vi "GUI_laptop v12.vi"() -> ()   [LabVIEW 2019]
uses:
  <vilib>/Math Plots/3D Math Plots/3D Scatter/3D Scatter XCtrl/3D Scatter.xctl
  <vilib>/Platform/TimedLoop/XDataNode/timing_clust.ctl
  <vilib>/Platform/TimedLoop/XDataNode/nitl_modes.ctl
  <vilib>/Platform/TimedLoop/XDataNode/wakeup.ctl
  <vilib>/Analysis/_algsub.llb/Real Vector Norm.vi
  <vilib>/Instr/_visa.llb/VISA Configure Serial Port (Instr).vi
  <vilib>/Utility/file.llb/Write Delimited Spreadsheet (DBL).vi
  <vilib>/Math Plots/3D Math Plots/3D Scatter/3D Scatter Datatype/Public/Plot Helper (Vector).vi
  <vilib>/platform/TimedLoop/XDataNode/XDataNode.xnode
  <vilib>/Platform/TimedLoop/XDataNode/XDNodeRunTimeDep.lvlib
  <vilib>/Analysis/NI_AALPro.lvlib
  <vilib>/Math Plots/3D Math Plots/3D Scatter/3D Scatter Datatype/3D Scatter Datatype.lvclass
panel:
  out "Numeric":i32
  out "send values":dbl[](array[numeric])
  out "Robot Feedback (xyz)":dbl[](array[numeric])
  in  "UDP Send":bool
  in  "UDP Recv":bool
  in  "L5 bound":dbl=1000.0
  in  "L4 bound (deg)":dbl=1000.0
  in  "L3 bound (mm)":dbl=1000.0
  in  "L2 bound (deg)":dbl=1000.0
  in  "L1 bound (deg)":dbl=1000.0
  in  "Joystick Type":dbl(ring) items=["Rigid Joystick", "Free Joystick"]
  out "Finished Late? [i-1]":bool
  in  "Epsilon":dbl=0.2
  out "3D Scatter":refnum<class "3D Plot Datatype.lvclass">[](xcontrol)
  out "Random Point":dbl[](array[numeric])
  out "Virtual Cursor":dbl[](array[numeric])
  out "Iteration Duration":i64
  in  "Num of Points":i32=10
  in  "z bound":dbl=2.0
  in  "y bound":dbl=5.0
  in  "x bound":dbl=5.0
  in  "Stop":bool
  in  "Round Decimals":dbl=2.0 format="%#_15g"
  in  "Save  Data":bool
  in  "Save Path":path
  in  "x speed":dbl=0.5
  in  "z speed":dbl=0.5
  in  "y speed":dbl=0.5
  out "error out":errorcluster
  in  "baud rate":u32=115200
  in  "VISA resource name":refnum<visa-resource-name>
  # "TODO: fix the bounds; currently bounds are arbitrary"
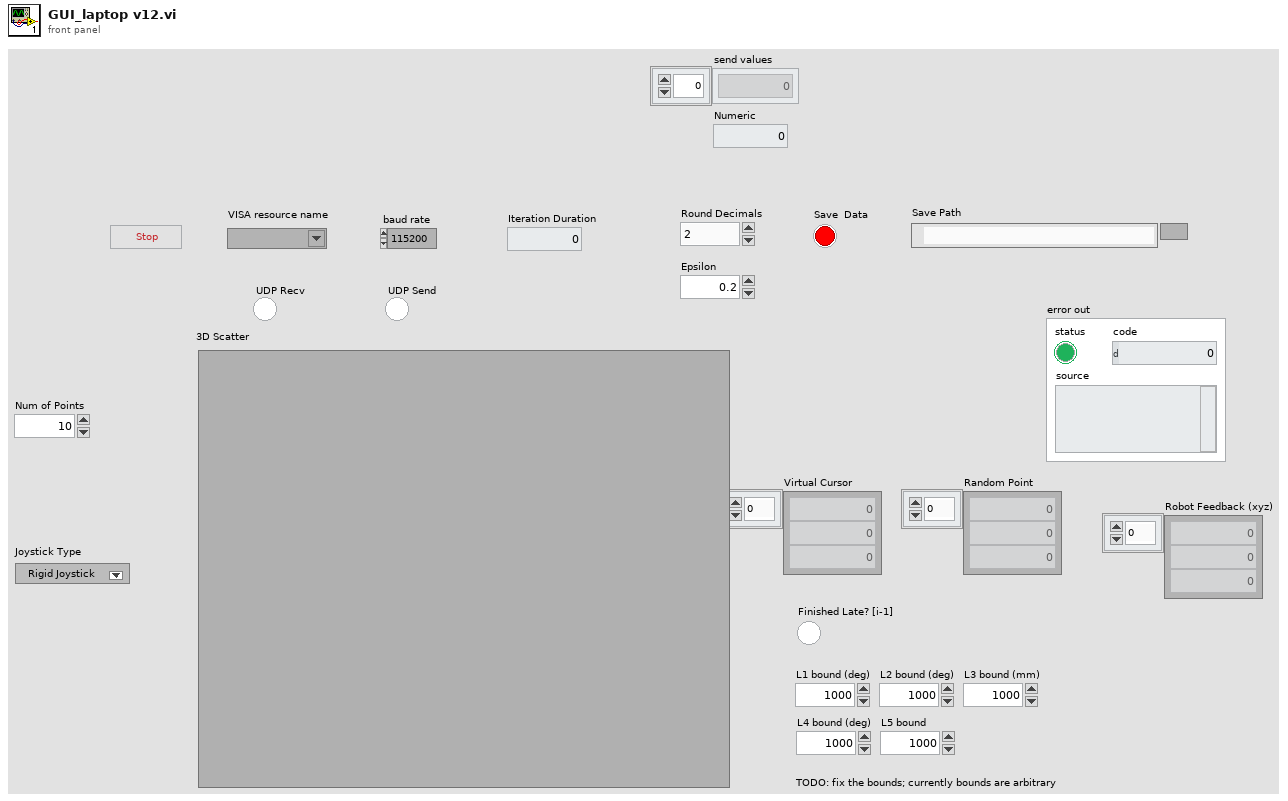
[diagram p1: front panel]
types:
  T1 = typedef "XDNodeRunTimeDep.lvlib/timing_clust.ctl" = cluster{"Expected End [f-1]":u64, "Actual End [f-1]":u64, "Finished Late? [f-1]":bool, "Expected End [i-1]":u64, "Actual End [i-1]":u64, "Finished Late? [i-1]":bool, "Expected Start [i]":u64, "Actual Start [i]":u64, "Expected Start [f]":u64, "Actual Start [f]":u64, "Source Name":string, "Structure Name":string, "Period":i64, "Deadline":i64, "Offset":i64, "Start":i64, "Priority":i32, "Timeout":i32, "Mode":T2, "Wakeup Reason":T3, "Error":errorcluster, "Source Type":string, "Secondary Source Type":string, "Global End Time":u64, "Global Start Time":u64, "Frame Duration":u64, "Iteration Duration":u64, "Assigned CPU":i32, "I/O Scan Engine Mode":u32}
  T2 = typedef "XDNodeRunTimeDep.lvlib/nitl_modes.ctl" = enum32{"No Change", "Process missed periods, maintain original phase", "Discard missed periods, maintain original phase", "Process missed periods, ignore original phase", "Discard missed periods, ignore original phase"}
  T3 = typedef "XDNodeRunTimeDep.lvlib/wakeup.ctl" = enum32{"Normal", "Aborted", "Asynchronous wakeup", "Timing source error", "Timed loop error", "Timeout"}
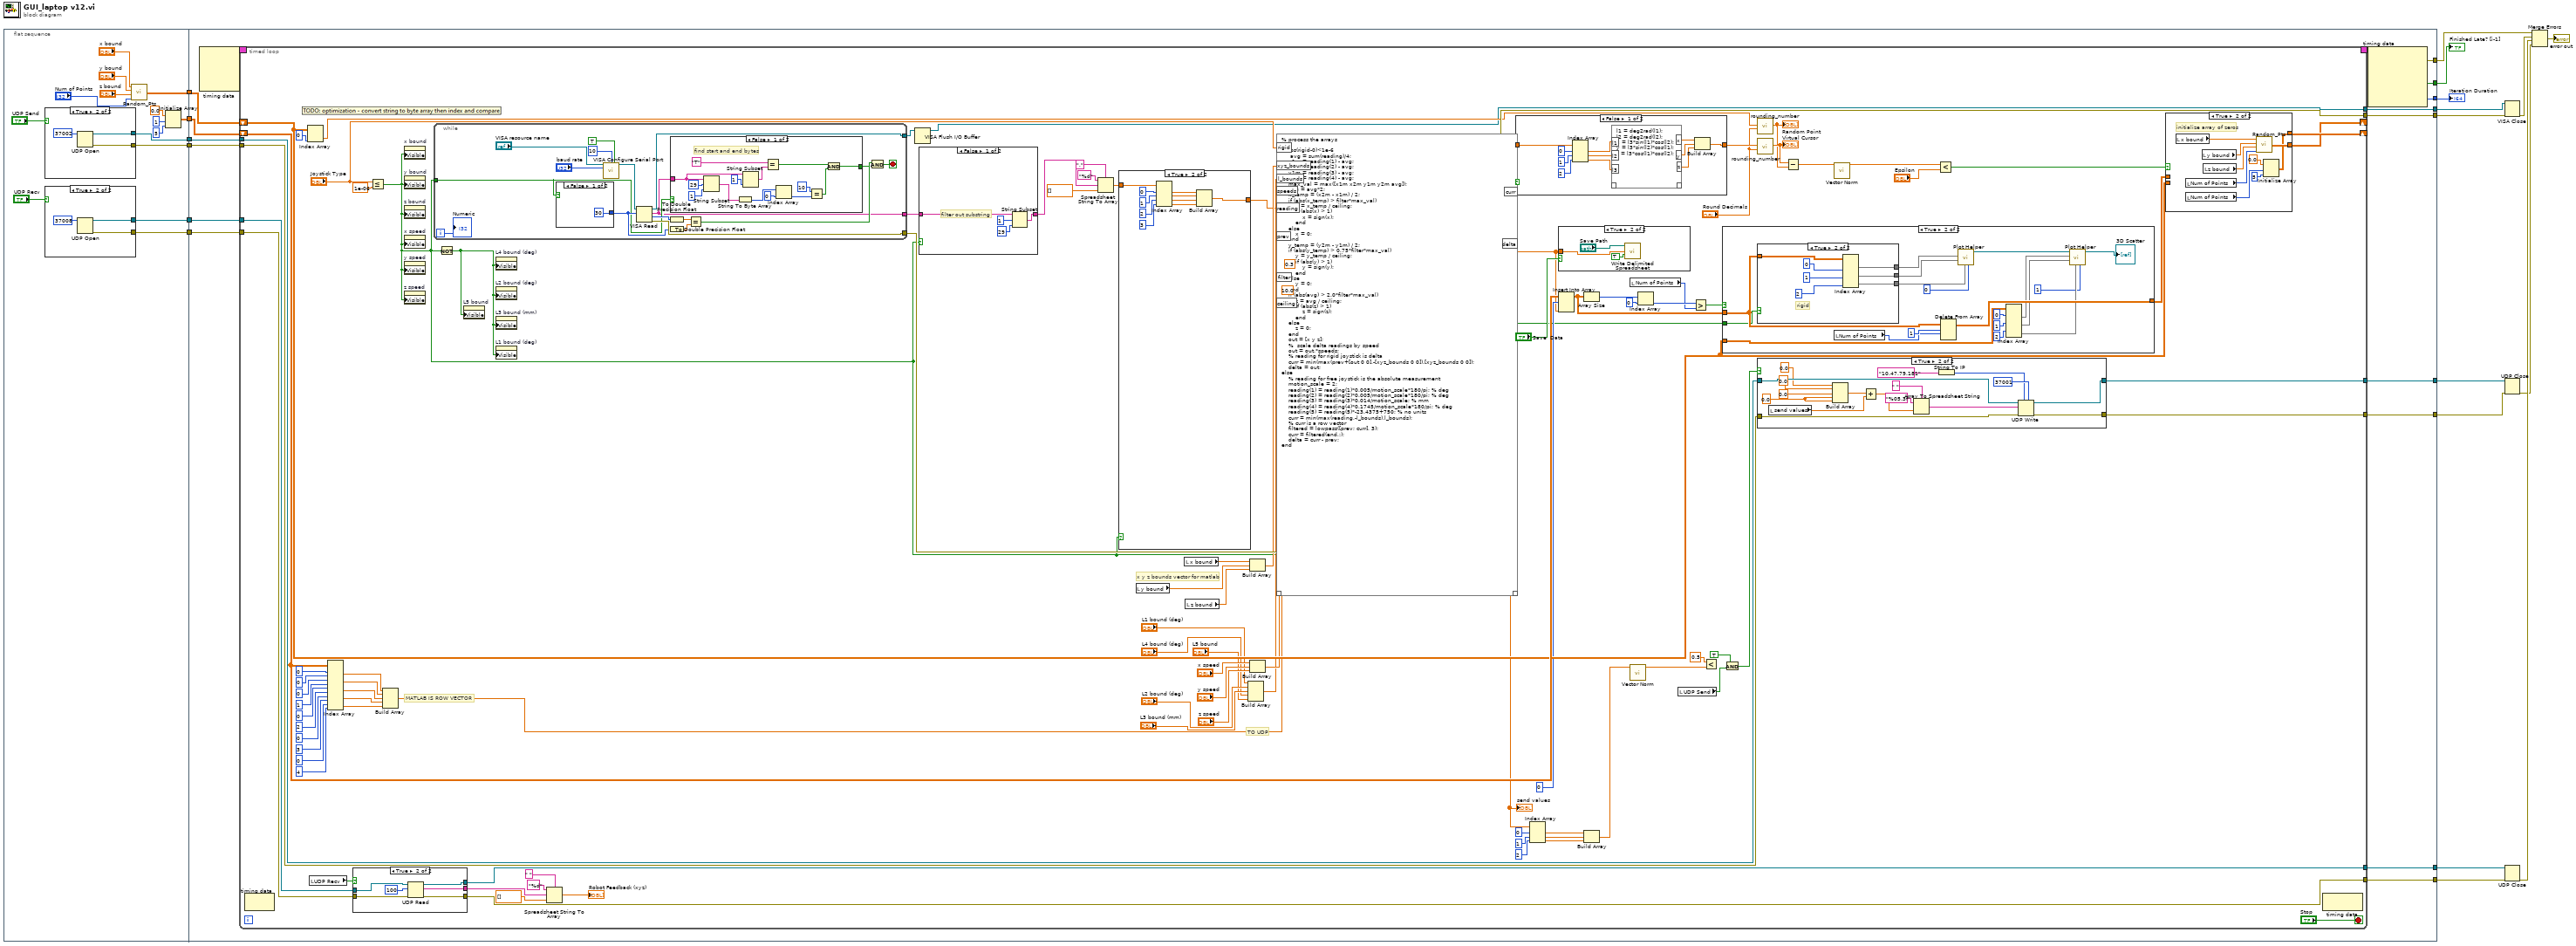
[diagram p0: block diagram]
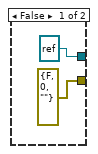
[diagram p2: hidden frame]
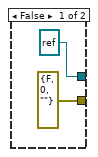
[diagram p3: hidden frame]
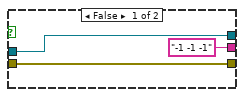
[diagram p5: hidden frame]
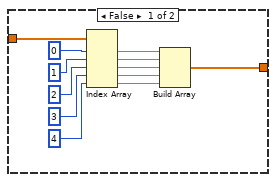
[diagram p9: hidden frame]
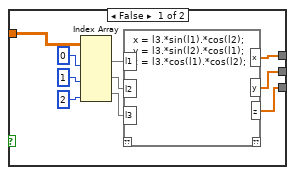
[diagram p12: hidden frame]
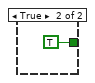
[diagram p13: hidden frame]
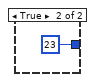
[diagram p14: hidden frame]
diagram:
  n1 = flat-sequence {
    tunnel: [w26] -> w15
    tunnel: [w30] -> w14
    tunnel: [w25] -> w13
    tunnel: [w24] -> w12
    tunnel: [w21] -> w11
    tunnel: [w20] -> w10
    tunnel: [w59] -> w19
    tunnel: [w58] -> w18
    tunnel: [w56] -> w9
    tunnel: [w54] -> w17
    tunnel: [w53] -> w16
    tunnel: w15 -> [w57]
    tunnel: w14 -> [w55]
    tunnel: w13 -> [w52]
    tunnel: w12 -> [w51]
    tunnel: w11 -> [w50]
    tunnel: w10 -> [w49]
    tunnel: [w48] -> w3
    tunnel: [w47] -> w8
    tunnel: [w46] -> w2
    tunnel: [w45] -> w1
    frame #0 {
      n2 = case shown="True" "UDP Send" {
        tunnel: [refnum<k16> refnum ("port") w38] -> w25
        tunnel: [errorcluster {"status"=FALSE, "code"=0, "source"=""} ("error out") w37] -> w20
        frame False {
        }
        frame True {
          n3 = UDP Open(11:u16 37002 ("port")) -> (port=w38:refnum<k16>, 0:w37:errorcluster)  [unwired: 4 in, 1 out]
        }
      }
      n4 = case shown="True" "UDP Recv" {
        tunnel: [refnum<k16> refnum ("port") w43] -> w24
        tunnel: [errorcluster {"status"=FALSE, "code"=0, "source"=""} ("error out") w42] -> w21
        frame False {
        }
        frame True {
          n5 = UDP Open(11:u16 37008 ("port")) -> (port=w43:refnum<k16>, 0:w42:errorcluster)  [unwired: 4 in, 1 out]
        }
      }
      n6 = call "Random_Pts.vi"("Num of Points"="Num of Points", "z bound"="z bound", "y bound"="y bound", "x bound"="x bound") -> ("appended array"=w30:dbl[][])
      n7 = Initialize Array(0.0 ("element"), 1 ("dimension size"), 5 ("dimension size")) -> (w26:dbl[][])
    }
    frame #1 {
      n8 = node-c288() -> (w61:T1)  [unwired: 4 in]
      n9 = timed-loop {
        tunnel: [w64] -> w59
        tunnel: [w158] -> w58
        shift-right: [w157] -> _
        shift-left: w57 -> [w156]
        timing: w61 -> [_]
        timing-out: [_] -> w60
        shift-right: [w152] -> _
        shift-left: w55 -> [w153]
        tunnel: w52 -> [w95]
        tunnel: w51 -> [w94]
        tunnel: w50 -> [w92]
        tunnel: w49 -> [w91]
        tunnel: [w90] -> w48
        tunnel: [w89] -> w47
        tunnel: [w88] -> w46
        tunnel: [w87] -> w45
        stop <- "Stop" stop-if-true
        # "TO UDP"
        # "MATLAB IS ROW VECTOR"
        # "x y z bounds vector for matlab"
        n10 = node-c288() -> ()  [unwired: 1 in, 1 out]
        n11 = Index Array(array=w153, index (col)=0 ("index (row)")) -> (element=w105:dbl[])  [unwired: 1 in]
        n12 = local read "UDP Recv"() -> (w93:bool)
        n13 = Index Array(array=w156, index (row) #1=0 ("disabled index (row)"), index (col) #1=0 ("disabled index (col)"), index (row) #2=0 ("disabled index (row)"), index (col) #2=1 ("disabled index (col)"), index (row) #3=0 ("disabled index (row)"), index (col) #3=2 ("disabled index (col)"), index (row) #4=0 ("disabled index (row)"), index (col) #4=3 ("disabled index (col)"), index (row) #5=0 ("disabled index (row)"), index (col) #5=4 ("disabled index (col)")) -> (element #1=w129:dbl, element #2=w128:dbl, element #3=w127:dbl, element #4=w113:dbl, element #5=w112:dbl)
        n14 = case shown="True" w93 {
          tunnel: w94 -> [w180 w187]
          tunnel: w92 -> [w181 w186]
          tunnel: [w181 w185] -> w90
          tunnel: [w180 w184] -> w88
          tunnel: ["-1 -1 -1" w182] -> w83
          frame False {
          }
          frame True {
            n15 = UDP Read(connection ID=w187, max size (548)=100, 8:w186) -> (data out=w182:string, error out=w185:errorcluster, 3:w184:refnum<k16>)  [unwired: 1 in, 2 out]
          }
        }
        n16 = Less Or Equal?(x="Joystick Type", y=1e-06) -> (x <= y?=w70:bool)
        n17 = Build Array(w129, w128, w127, w113, w112) -> (w126:dbl[])
        n18 = property on="x bound" class="DigNum (strict)"("Visible"=w70) -> ()  [unwired: 2 in, 2 out]
        n19 = property on="y bound" class="DigNum (strict)"("Visible"=w70) -> ()  [unwired: 2 in, 2 out]
        n20 = property on="z bound" class="DigNum (strict)"("Visible"=w70) -> ()  [unwired: 2 in, 2 out]
        n21 = property on="x speed" class="DigNum (strict)"("Visible"=w70) -> ()  [unwired: 2 in, 2 out]
        n22 = property on="y speed" class="DigNum (strict)"("Visible"=w70) -> ()  [unwired: 2 in, 2 out]
        n23 = property on="z speed" class="DigNum (strict)"("Visible"=w70) -> ()  [unwired: 2 in, 2 out]
        n24 = while {
          tunnel: [w279] -> w107
          tunnel: [w292] -> w158
          tunnel: [w286] -> w65
          tunnel: w70 -> [w280]
          i -> [w278]
          stop <- w282 stop-if-true
          n25 = case shown="False" w280 {
            tunnel: [30 u32 23 ("byte count")] -> w285
            frame False {
            }
            frame True {
            }
          }
          n26 = call-poly "VISA Configure Serial Port"("VISA resource name"="VISA resource name", "termination char\n(0xA = '\\n' = LF)"=u8 10 ("termination char\n(0xA = '\\n' = LF)"), "Enable Termination\nChar (T)"=TRUE ("Enable Termination\nChar (T)"), "baud rate (9600)"="baud rate") -> ("VISA resource name out"=w287:refnum<visa-resource-name>)  [unwired: 10 in, 1 out]
          n27 = VISA Read(VISA resource name=w287, byte count=w285) -> (VISA resource name out=w286:refnum<visa-resource-name>, read buffer=w279:string, return count=w294:u32, error out=w292:errorcluster)  [unwired: 1 in]
          n28 = To Double Precision Float(number=w294) -> (double precision float=w293:dbl)
          n29 = To Double Precision Float(number=w285) -> (double precision float=w284:dbl)
          n30 = case shown="False" w280 {
            tunnel: [w301 TRUE] -> w281
            tunnel: w279 -> [w304 _]
            frame False {
              # "find start and end bytes"
              n31 = String Subset(string=w304, offset (0)=29, length (rest)=1) -> (substring=w299:string)
              n32 = String To Byte Array(string=w299) -> (unsigned byte array=w298:u8[])
              n33 = String Subset(string=w304, length (rest)=1) -> (substring=w307:string)  [unwired: 1 in]
              n34 = Equal?(x="T", y=w307) -> (x = y?=w303:bool)
              n35 = Index Array(array=w298, index=0) -> (element=w296:u8)
              n36 = Equal?(x=10, y=w296) -> (x = y?=w302:bool)
              n37 = And(x=w303, y=w302) -> (x .and. y?=w301:bool)
            }
            frame True {
            }
          }
          n38 = Equal?(x=w293, y=w284) -> (x = y?=w283:bool)
          n39 = And(x=w283, y=w281) -> (x .and. y?=w282:bool)
          "Numeric" <- w278
        }
        n40 = Not(x=w70) -> (.not. x?=w69:bool)
        n41 = property on="L5 bound" class="DigNum (strict)"("Visible"=w69) -> ()  [unwired: 2 in, 2 out]
        n42 = property on="L4 bound (deg)" class="DigNum (strict)"("Visible"=w69) -> ()  [unwired: 2 in, 2 out]
        n43 = property on="L2 bound (deg)" class="DigNum (strict)"("Visible"=w69) -> ()  [unwired: 2 in, 2 out]
        n44 = property on="L3 bound (mm)" class="DigNum (strict)"("Visible"=w69) -> ()  [unwired: 2 in, 2 out]
        n45 = property on="L1 bound (deg)" class="DigNum (strict)"("Visible"=w69) -> ()  [unwired: 2 in, 2 out]
        n46 = Spreadsheet String To Array(delimiter (Tab)=" ", format string="%d", spreadsheet string=w83, array type (2D Dbl)=dbl[] []) -> (array=→"Robot Feedback (xyz)":dbl[])
        n47 = VISA Flush I/O Buffer(VISA resource name=w65) -> (VISA resource name out=w64:refnum<visa-resource-name>)  [unwired: 2 in, 1 out]
        n48 = case shown="False" w70 {
          tunnel: w107 -> [w205 w206]
          tunnel: [w202 w206] -> w106
          frame False {
            # "filter out substring"
            n49 = String Subset(string=w205, offset (0)=1, length (rest)=29) -> (substring=w202:string)
          }
          frame True {
          }
        }
        n50 = Spreadsheet String To Array(delimiter (Tab)=",", format string="%d", spreadsheet string=w106, array type (2D Dbl)=dbl[] []) -> (array=w109:dbl[])
        n51 = case shown="True" w70 {
          tunnel: w109 -> [w207 w222]
          tunnel: [w212 w221] -> w108
          frame False {
            n52 = Index Array(array=w207, index #1=0 ("Plot ID"), index #2=1 ("Plot ID"), index #3=2 ("Plot ID"), index #4=3 ("Plot ID"), index #5=4 ("Plot ID")) -> (element #1=w215:dbl, element #2=w214:dbl, element #3=w213:dbl, element #4=w209:dbl, element #5=w208:dbl)
            n53 = Build Array(w215, w214, w213, w209, w208) -> (w212:dbl[])
          }
          frame True {
            n54 = Index Array(array=w222, index #1=0 ("Plot ID"), index #2=1 ("Plot ID"), index #3=2 ("Plot ID"), index #4=3 ("index")) -> (element #1=w225:dbl, element #2=w224:dbl, element #3=w223:dbl, element #4=w219:dbl)
            n55 = Build Array(w225, w224, w223, w219) -> (w221:dbl[])
          }
        }
        n56 = local read "y bound"() -> (w131:dbl)
        n57 = local read "x bound"() -> (w132:dbl)
        n58 = local read "z bound"() -> (w130:dbl)
        n59 = Build Array("L1 bound (deg)", "L2 bound (deg)", "L3 bound (mm)", "L4 bound (deg)", "L5 bound") -> (w120:dbl[])
        n60 = Build Array(w132, w131, w130) -> (w124:dbl[])
        n61 = Build Array("x speed", "y speed", "z speed") -> (w125:dbl[])
        n62 = script code="% process the arrays\n\nif abs(rigid-0)<1e-6\n     avg = sum(reading)/4;\n    x1m = reading(1) - avg;\n    x2m = reading(2) - avg;\n    y1m = reading(3) - avg;\n    y2m = reading(4) - avg;\n    max_val = max([x1m x2m y1m y2m avg]);\n    avg = avg*2;\n    x_temp = (x2m - x1m) / 2;\n    if (abs(x_temp) > filter*max_val)\n        x = x_temp / ceiling;\n        if (abs(x) > 1)\n            x = sign(x);\n        end\n    else\n        x = 0;\n    end\n    y_temp = (y2m - y1m) / 2;\n    if (abs(y_temp) > 0.75*filter*max_val)\n        y = y_temp / ceiling;\n        if (abs(y) > 1)\n            y = sign(y);\n        end\n    else\n        y = 0;\n    end\n    if (abs(avg) > 2.0*filter*max_val)\n        z = avg / ceiling;\n        if (abs(z) > 1)\n            z = sign(z);\n        end\n    else\n        z = 0;\n    end\n    out = [x y z];\n    %  scale delta readings by speed\n    out = out.*speeds;\n    % reading for rigid joystick is delta\n    curr = min(max(prev+[out 0 0],-[xyz_bounds 0 0]),[xyz_bounds 0 0]);\n    delta = out;\nelse\n    % reading for free joystick is the absolute measurement\n    motion_scale = 2;\n    reading(1) = reading(1)*0.005/motion_scale*180/pi; % deg\n    reading(2) = reading(2)*0.005/motion_scale*180/pi; % deg\n    reading(3) = reading(3)*0.014/motion_scale; % mm\n    reading(4) = reading(4)*0.1745/motion_scale*180/pi; % deg\n    reading(5) = reading(5)*-23.4375+750; % no units\n    curr = min(max(reading,-l_bounds),l_bounds);\n    % curr is a row vector\n    filtered = lowpass([prev; curr], 3);\n    curr = filtered(end,:);\n    delta = curr - prev;\nend"("xyz_bounds"=w124, "speeds"=w125, "reading"=w108, "prev"=w126, "rigid"="Joystick Type", "l_bounds"=w120, "filter"=0.3 ("Real"), "ceiling"=10.0 ("Real")) -> ("curr"=w66:dbl[], "delta"=w62:dbl[])  [unwired: 1 in, 1 out]
        "send values" <- w62
        n63 = case shown="False" w70 {
          tunnel: w66 -> [w236 w240]
          tunnel: [w229 w240] -> w154
          frame False {
            n64 = Index Array(array=w236, index #1=0 ("Plot ID"), index #2=1 ("Plot ID"), index #3=2 ("Plot ID")) -> (element #1=w235:dbl, element #2=w234:dbl, element #3=w233:dbl)
            n65 = script code="l1 = deg2rad(l1);\nl2 = deg2rad(l2);\nx = l3*sin(l1)*cos(l2);\ny = l3*sin(l2)*cos(l1);\nz = l3*cos(l1)*cos(l2);"("l1"=w235, "l2"=w234, "l3"=w233) -> ("x"=w232:dbl, "y"=w231:dbl, "z"=w230:dbl)  [unwired: 1 in, 1 out]
            n66 = Build Array(w232, w231, w230) -> (w229:dbl[])
          }
          frame True {
          }
        }
        n67 = Index Array(array=w62, index #1=0 ("disabled index (col)"), index #2=1 ("disabled index (col)"), index #3=2 ("disabled index (col)")) -> (element #1=w74:dbl, element #2=w73:dbl, element #3=w72:dbl)
        n68 = case shown="True" "Save  Data" {
          tunnel: w66 -> [_ w188]
          frame False {
          }
          frame True {
            n69 = call-poly <vilib>:"Write Delimited Spreadsheet.vi"("file path (dialog if empty)"="Save Path", "1D data"=w188, "append to file? (new file:F)"=TRUE) -> ()  [unwired: 11 in, 2 out]
          }
        }
        n70 = Insert Into Array(array=w156, index (row)=0, new element=w66) -> (w137:dbl[][])  [unwired: 1 in]
        n71 = Array Size(array=w137) -> (size(s)=w139:i32[])
        n72 = Build Array(w74, w73, w72) -> (w71:dbl[])
        n73 = local read "Num of Points"() -> (w138:i32)
        n74 = call-poly <vilib>:"Vector Norm.vi"("Input Vector"=w71) -> ("norm"=w81:dbl)  [unwired: 9 in, 1 out]
        n75 = Index Array(array=w139, index=0) -> (element=w140:i32)
        n76 = local read "UDP Send"() -> (w79:bool)
        n77 = Greater?(x=w140, y=w138) -> (0:w136:bool)
        n78 = Less?(x=0.5, y=w81) -> ()  [unwired: 1 out]
        n79 = case shown="True" w136 {
          tunnel: w137 -> [w241 w259]
          tunnel: [w241 w258] -> w155
          tunnel: w153 -> [_ w257]
          tunnel: w70 -> [_ w242]
          frame False {
          }
          frame True {
            n80 = case shown="True" w242 {
              tunnel: w259 -> [w270 w274]
              tunnel: [w261 w273] -> w248
              tunnel: [w262 w272] -> w247
              tunnel: [w263 w271] -> w246
              frame False {
                n81 = Index Array(array=w270, index (col) #1=0 ("Plot ID"), index (col) #2=1 ("Plot ID"), index (col) #3=2 ("Plot ID")) -> (element #1=w266:dbl[], element #2=w265:dbl[], element #3=w264:dbl[])  [unwired: 3 in]
                n82 = script code="x = l3.*sin(l1).*cos(l2);\ny = l3.*sin(l2).*cos(l1);\nz = l3.*cos(l1).*cos(l2);"("l1"=w266, "l2"=w265, "l3"=w264) -> ("x"=w261:dbl[], "y"=w262:dbl[], "z"=w263:dbl[])  [unwired: 1 in, 1 out]
              }
              frame True {
                # "rigid"
                n83 = Index Array(array=w274, index (col) #1=0 ("disabled index (col)"), index (col) #2=1 ("index (col)"), index (col) #3=2 ("index (col)")) -> (element #1=w273:dbl[], element #2=w272:dbl[], element #3=w271:dbl[])  [unwired: 3 in]
              }
            }
            n84 = local read "Num of Points"() -> (w256:i32)
            n85 = Delete From Array(array=w259, length=1, index (row)=w256) -> (array with subset deleted=w258:dbl[][])  [unwired: 1 in, 1 out]
            n86 = call-poly <vilib>:"Plot Helper.vi"("Plot ID"=0, "z vector"=w246, "y vector"=w247, "x vector"=w248) -> ("3D Plot lvclass Array out"=w250:refnum<class "3D Plot Datatype.lvclass">[])  [unwired: 2 in, 5 out]
            n87 = Index Array(array=w257, index (row) #1=0 ("index (row)"), index (row) #2=1 ("index (row)"), index (row) #3=2 ("index (row)")) -> (element #1=w254:dbl[], element #2=w253:dbl[], element #3=w252:dbl[])  [unwired: 3 in]
            n88 = call-poly <vilib>:"Plot Helper.vi"("Plot ID"=1, "z vector"=w252, "y vector"=w253, "x vector"=w254, "3D Plot lvclass Array in"=w250) -> ("3D Plot lvclass Array out"=→"3D Scatter":refnum<class "3D Plot Datatype.lvclass">[])  [unwired: 1 in, 5 out]
          }
        }
        n89 = And(x=TRUE, y=w79) -> (x .and. y?=w78:bool)
        n90 = call "rounding_number.vi"("power of ten"="Round Decimals", "Array"=w105) -> ("rounded"=w101:dbl[])  [unwired: 9 in]
        "Random Point" <- w101
        n91 = call "rounding_number.vi"("power of ten"="Round Decimals", "Array"=w154) -> ("rounded"=w102:dbl[])  [unwired: 9 in]
        "Virtual Cursor" <- w102
        n92 = case shown="True" w78 {
          tunnel: w95 -> [w160 w178]
          tunnel: w91 -> [w161 w174]
          tunnel: [w161 w170] -> w89
          tunnel: [w160 w169] -> w87
          frame False {
          }
          frame True {
            w168 = 0.0 ("element")
            n93 = local read "send values"() -> (w166:dbl[])
            n94 = Build Array(0.0 ("element"), 0.0 ("element"), 0.0 ("element"), w168, w168) -> (w167:dbl[])
            n95 = Add(x=w167, y=w166) -> (x+y=w165:dbl[])
            n96 = Array To Spreadsheet String(delimiter (Tab)=" ", array=w165, 3:"%05.3f" ("format string")) -> (spreadsheet string=w175:string)
            n97 = String To IP(1:"10.47.79.181" ("name")) -> (0:w172:u32)
            n98 = UDP Write(address=w172, port or service name=u16 37001, connection ID=w178, data in=w175, 8:w174) -> (error out=w170:errorcluster, 3:w169:refnum<k16>)  [unwired: 1 in]
          }
        }
        n99 = Subtract(x=w102, y=w101) -> (x-y=w100:dbl[])
        n100 = call-poly <vilib>:"Vector Norm.vi"("Input Vector"=w100) -> ("norm"=w99:dbl)  [unwired: 9 in, 1 out]
        n101 = Less?(x=w99, y="Epsilon") -> (x < y?=w97:bool)
        n102 = case shown="True" w97 {
          tunnel: w153 -> [w192 _]
          tunnel: [w192 w197] -> w152
          tunnel: w155 -> [w191 _]
          tunnel: [w191 w193] -> w157
          frame False {
          }
          frame True {
            # "initialize array of zeros"
            n103 = local read "x bound"() -> (w201:dbl)
            n104 = local read "Num of Points"() -> (w198:i32)
            n105 = local read "Num of Points"() -> (w195:i32)
            n106 = local read "y bound"() -> (w200:dbl)
            n107 = local read "z bound"() -> (w199:dbl)
            n108 = call "Random_Pts.vi"("Num of Points"=w198, "z bound"=w199, "y bound"=w200, "x bound"=w201) -> ("appended array"=w197:dbl[][])
            n109 = Initialize Array(0.0 ("element"), w195, 5 ("dimension size")) -> (w193:dbl[][])
          }
        }
        n110 = node-c288() -> ()  [unwired: 1 in, 1 out]
      }
      n111 = node-c288(w60) -> (w56:errorcluster, w53:bool, w54:i64)  [unwired: 3 out]
    }
  }
  n112 = VISA Close(VISA resource name=w19, error in (no error)=w18) -> (error out=w7:errorcluster)
  n113 = UDP Close(connection ID=w1, 8:w8) -> (error out=w5:errorcluster)  [unwired: 1 out]
  n114 = UDP Close(connection ID=w2, 8:w3) -> (error out=w6:errorcluster)  [unwired: 1 out]
  n115 = Merge Errors(w9, w7, w6, w5) -> (→"error out":errorcluster)
  "Iteration Duration" <- w17
  "Finished Late? [i-1]" <- w16
